vi "set_result.vi"(11 "error in":errorcluster) -> (2 "string":string, 3 "font color":u32)   [LabVIEW 2020]
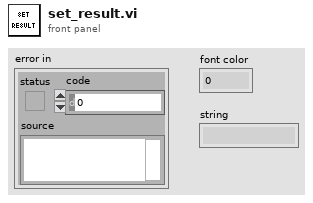
[diagram p1: front panel]
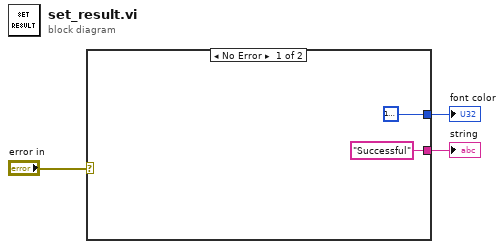
[diagram p0: block diagram]
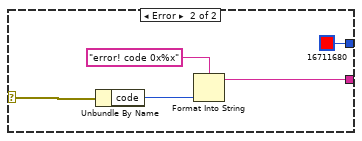
[diagram p2: hidden frame]
diagram:
  n1 = case shown="No Error" "error in" {
    selector: "error in" -> [_ w6]
    tunnel: [u32 16777228 u32 16711680] -> w3
    tunnel: ["Successful" w9] -> w2
    frame No Error {
    }
    frame Error {
      n2 = Unbundle By Name(w6) -> ("code"=w7:i32)
      n3 = Format Into String(format string="error! code 0x%x", w7) -> (resulting string=w9:string)  [unwired: 2 in, 1 out]
    }
  }
  "font color" <- w3
  "string" <- w2
